vi "Finalize.vi"(8 "error in":errorcluster, 11 "Plugin in":refnum<class "CSV Export.lvclass">) -> (0 "error out":errorcluster, 3 "Plugin out":refnum<class "CSV Export.lvclass">)   [LabVIEW 2022 SP3, in "CSV Export.lvlib" / "CSV Export.lvclass"]
uses:
  CSV Export.lvclass
  C:/Program Files/National Instruments/LabVIEW 2022/vi.lib/FlexLogger/SDK/PluginSDK.lvlibp/PEFClasses/SDK/Processing Element/Processing Element.lvclass
  <vilib>/FlexLogger/SDK/PluginSDK.lvlibp/PEFClasses/SDK/Processing Element/Read System Interface.vi
  <vilib>/FlexLogger/SDK/PluginSDK.lvlibp/PEFClasses/SDK/Processing Element/Read Alias.vi
  Global.vi
  <vilib>/FlexLogger/SDK/PluginSDK.lvlibp/PEFClasses/SDK/System Interface/System Interface.lvclass
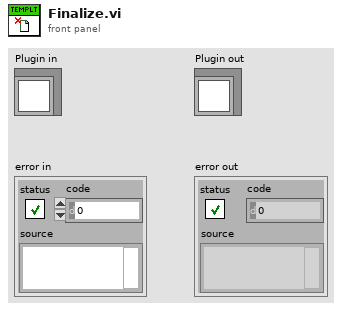
[diagram p1: front panel]
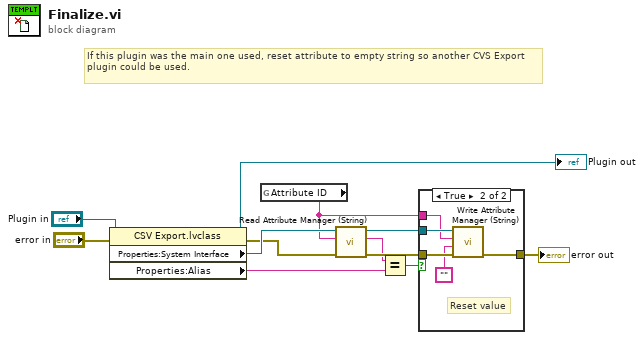
[diagram p0: block diagram]
diagram:
  # "If this plugin was the main one used, reset attribute to empty string so another CVS Export plugin could be used."
  n1 = property class="CSV Export.lvclass"(reference="Plugin in", error in="error in") -> (reference out=→"Plugin out":refnum<class "CSV Export.lvclass">, error out=w11:errorcluster, "Properties:System Interface"=w12:refnum<class "System Interface.lvclass">, "Properties:Alias"=w4:string)
  n2 = global read "Global.vi" "Attribute ID"() -> (w8:string)
  n3 = call-dynamic "Read Attribute Manager (String).vi"("error in (no error)"=w11, "Attribute ID"=w8, "System Interface in"=w12) -> ("error out"=w9:errorcluster, "Attrib Val"=w5:string, "System Interface out"=w10:refnum<class "System Interface.lvclass">)  [unwired: 5 in, 1 out]
  n4 = Equal?(x=w5, y=w4) -> (x = y?=w3:bool)
  n5 = case shown="True" w3 {
    tunnel: w10 -> [_ w18]
    tunnel: w9 -> [w13 w17]
    tunnel: w8 -> [_ w16]
    tunnel: [w13 w15] -> w2
    frame False {
      # "Not the same instance, so don't cvhange value"
    }
    frame True {
      # "Reset value"
      n6 = call-dynamic "Write Attribute Manager (String).vi"("error in (no error)"=w17, "Attribute Value"="", "Attribute ID"=w16, "System Interface in"=w18) -> ("error out"=w15:errorcluster)  [unwired: 5 in, 2 out]
    }
  }
  "error out" <- w2
